vi "ScreenCoordinates.vi"(8 "error in (no error)":errorcluster, 9 "Left Coordinate":i16, 10 "Top Coordinate":i16, 11 "ThisVI":refnum<vi>) -> (0 "error out":errorcluster, 3 "reference out":refnum<vi>)   [LabVIEW 2021]
doc: "Sets screen position for DUT Information dialog and result banners."
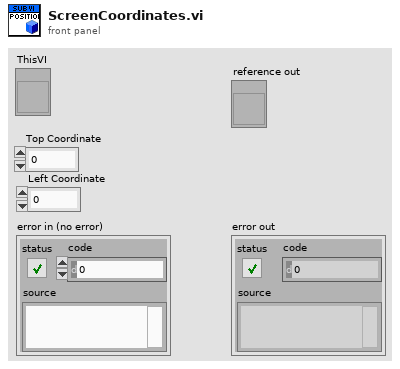
[diagram p1: front panel]
types:
  T1 = typedef "LVRectTypeDef.ctl" = cluster{"Left":i16, "Top":i16, "Right":i16, "Bottom":i16}
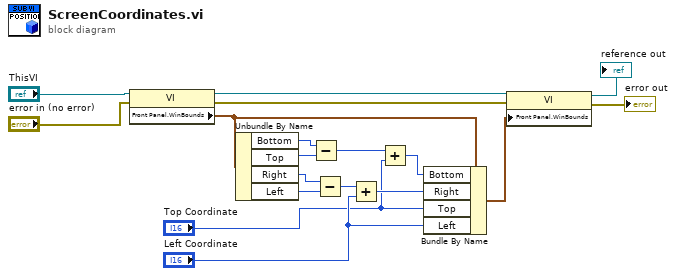
[diagram p0: block diagram]
diagram:
  n1 = property on="Property Node" class="VI"(reference="ThisVI", error in="error in (no error)") -> (reference out=w13:refnum<vi>, error out=w14:errorcluster, "Front Panel.WinBounds"=w15:T1)
  n2 = Unbundle By Name(w15) -> ("Bottom"=w7:i16, "Top"=w6:i16, "Right"=w12:i16, "Left"=w11:i16)
  n3 = Subtract(x=w7, y=w6) -> (x-y=w5:i16)
  n4 = Subtract(x=w12, y=w11) -> (x-y=w10:i16)
  n5 = Add(x=w10, y="Left Coordinate") -> (x+y=w8:i16)
  n6 = Add(x=w5, y="Top Coordinate") -> (x+y=w3:i16)
  n7 = Bundle By Name(cluster=w15, "Bottom"=w3, "Right"=w8, "Top"="Top Coordinate", "Left"="Left Coordinate") -> (w18:T1)
  n8 = property on="Property Node" class="VI"(reference=w13, error in=w14, "Front Panel.WinBounds"=w18) -> (reference out=→"reference out":refnum<vi>, error out=→"error out":errorcluster)
